vi "Example 2 Transient.vi"() -> ()   [LabVIEW 2015]
panel:
  out "time string 2":string
  out "time string":string
  in  "RANDOM":bool
  out "size(s)":i32
  out "Numeric":i32
  in  "Tab Control":enum32{"Page 1", "Page 2"}(tab)
  in  "no":bool
  in  "yes":bool
  in  "Memory SAVE":u16(ring)=3 items=["1", "2", "3", "4"]
  in  "message":string="Do you want store\n transient values"
  out "Model and SW rev,":string
  out "Array":string[](array[string])=["0,\"No error\""]
  in  "Tab Control 2":enum32{"INTERFACE", "TRANSIENT"}(tab)
  in  "Setting OK":bool
  in  "VISA":refnum<visa-resource-name>="COM1"
  in  "Baud Rate":i32(ring)=3 items=["1200", "2400", "4800", "9600", "19200", "38400", "57600", "115200"]
  in  "Address":i16=6
  in  "Voltage Limit at start":dbl=1.0 format="%.4f"
  in  "Current Limit at start":dbl=1.0 format="%.4f"
  in  "Reset (T)":bool
  out "Communication":bool=TRUE
  out "Appl. Rev":string
  in  "SCALE x":i8(slide)=1 scale=1.0..5.0
  in  "Tab Control 3":enum32{"Page 1", "Page 2"}(tab)
  in  "Max Element":i32=12
  out "Time/Dwell string [S]":string="0.97,0.90,0.45,0.31,0.84,0.30,0.65,0.95,0.00,0.05,0.72,0.12\r\n"
  out "Value string":string="7.93,8.01,0.22,1.41,9.70,1.73,7.77,7.95,7.10,1.88,5.55,1.76\r\n"
  in  "Max Time":dbl=1.0
  in  "Max Value":dbl=10.0
  out "Triggering value":dbl=0.9353250304502314
  in  "Step &\nCounter":cluster{"Step":u16, "Counter":dbl}={"Step"=1, "Counter"=1.0} {"Counter" min=1.0 max=9999.0 step=1.0; "Step" items=["ONCE", "AUTO"]}
  in  "Continius":u16(ring) caption="Continues (Default:0)" items=["0", "1"]
  out "Condition Setting":bool=TRUE
  in  "MODE":T1 caption="Cluster 1" {"Trans Mode (None)" items=["NONE", "FIX", "LIST", "WAVE"]; "Mode (V/I)" items=["VOLTAGE", "CURRENT"]}
  in  "Values":T2={"Value string"="001.00,003.00,002.00,004.00,003.00", "Time/Dwell string [S]"="0.100,0.100,0.100,0.100,0.100", "Triggering value "=0.0}
  out "Error":string
  out "READ VALUE":dbl format="%.4f"
  in  "dt Resolution":dbl=0.025 min=0.0 max=1.0 step=0.001
  in  "INIT":bool
  in  "Read SET/MEAS":bool=TRUE
  in  "ABORT":bool
  out "Waveform Graph":dynamicdata(graph)=[{"t0"=timestamp(0 s since 1904-01-01), "dt"=1.0, "Y"=[-0.05, -0.05, -0.05, -0.05, -0.05]}, {"t0"=timestamp(0 s since 1904-01-01), "dt"=0.02, "Y"=[7.81, 7.81, 7.81, 7.81, 7.81, 7.81, 7.81, 7.81, 7.81, 7.81, 7.81, 7.81, 7.81, 7.81, 7.81, 7.81, 7.81, 7.81, 7.81, 7.81, 7.81, 7.81, 7.81, 7.81, 7.81, 7.81, 7.81, 7.81, 7.81, 7.81, 7.81, 7.81, 7.81, 7.81, 7.81, 7.81, 7.81, 7.81, 7.81, 7.81, 7.81, 7.81, 7.81, 7.81, 7.81, 7.81, 7.81, 7.81, 7.81, 7.81, 7.81, 7.81, 7.81, 7.81, 7.81, 7.81, 7.81, 7.81, 7.81, 7.81, 7.81, 7.81, 7.81, 7.81, 7.81, 7.81, 7.81, 7.81, 7.81, 7.81, 7.81, 7.81, 7.81, 7.81, 7.81, 7.81, 7.81, 7.81, 7.81, 7.81, 7.81, 7.81, 7.81, 7.81, 7.81, 7.81, 7.81, 7.81, 7.81, 7.81, 7.81, 7.81, 7.81, 7.81, 7.81, 7.81, 7.81, 7.81, 7.81, 7.81, 7.81, 7.81, 7.81, 7.81, 7.81, 7.81, 7.81, 7.81, 7.81, 7.81, 7.81, 7.81, 7.81, 7.81, 7.81, 7.81, 7.81, 7.81, 7.81, 7.81, 7.81, 7.81, 7.81, 7.81, 7.81, 7.81, 7.81, 7.81, 7.81, 7.81, 7.81, 7.81, 7.81, 7.81, 7.81, 7.81, 7.81, 7.81, 7.81, 7.81, 7.81, 7.81, 7.81, 7.81, 7.81, 7.81, 7.81, 7.81, 7.81, 7.81, 7.81, 7.81, 7.81, 7.81, 7.81, 7.81, 7.81, 7.81, 7.81, 7.81, 7.81, 7.81, 7.81, 7.81, 7.81, 7.81, 7.81, 7.81, 7.81, 7.81, 7.81, 7.81, 7.81, 7.81, 7.81, 7.81, 7.81, 7.81, 7.81, 7.81]}]
  in  "Trig":bool
  in  "stop":bool
  in  "LOAD":enum32{"1", "2", "3", "4"}(radio)
  in  "STORe":enum32{"1", "2", "3", "4"}(radio)
  out "error out":errorcluster
  # "Configurate transient\nparameters"
  # "Z+ POWER SUPPLY"
  # "Set required interface and output parameters."
  # "PS Communication Language - SCPI"
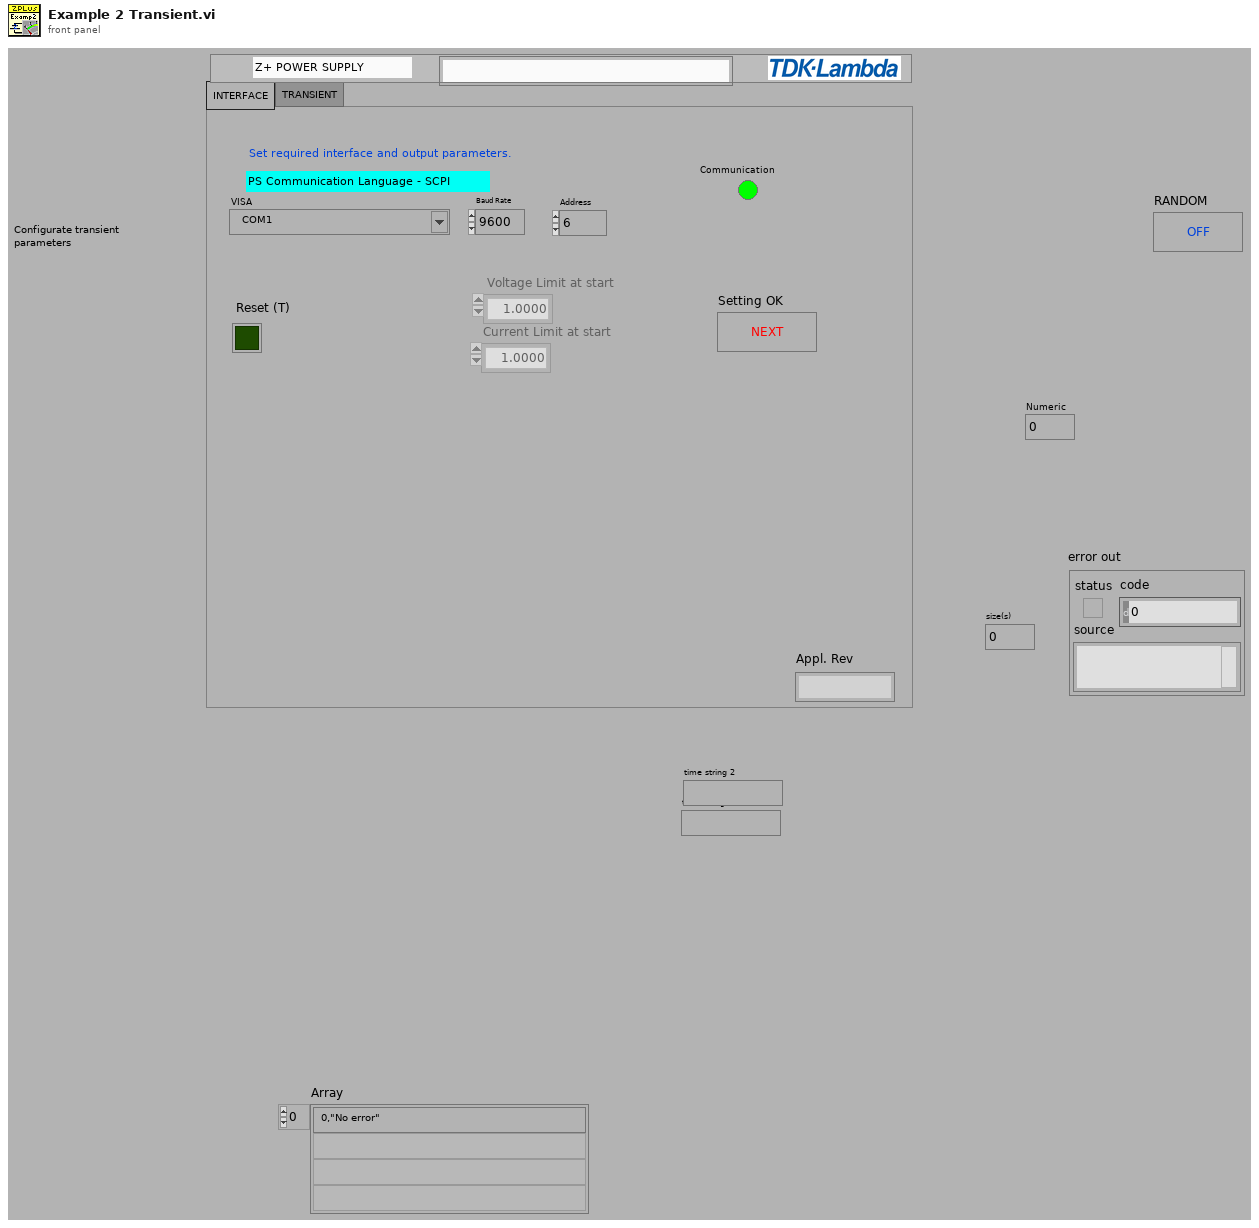
[diagram p1: front panel]
types:
  T1 = cluster{"Mode (V/I)":u16, "Trans Mode (None)":u16}
  T2 = cluster{"Value string":string, "Time/Dwell string [S]":string, "Triggering value ":dbl}
  T3 = enum8{"Enabled", "Disabled", "Disabled and Grayed Out"}
  T4 = cluster{"Response":string, "Response":string, "Triggering value (for fix)":dbl}
  T5 = cluster{"Value string":bool, "Time/Dwell string [S]":bool, "Triggering value ":bool}
  T6 = cluster{"Mode (V/I)":bool, "Trans Mode (None)":bool}
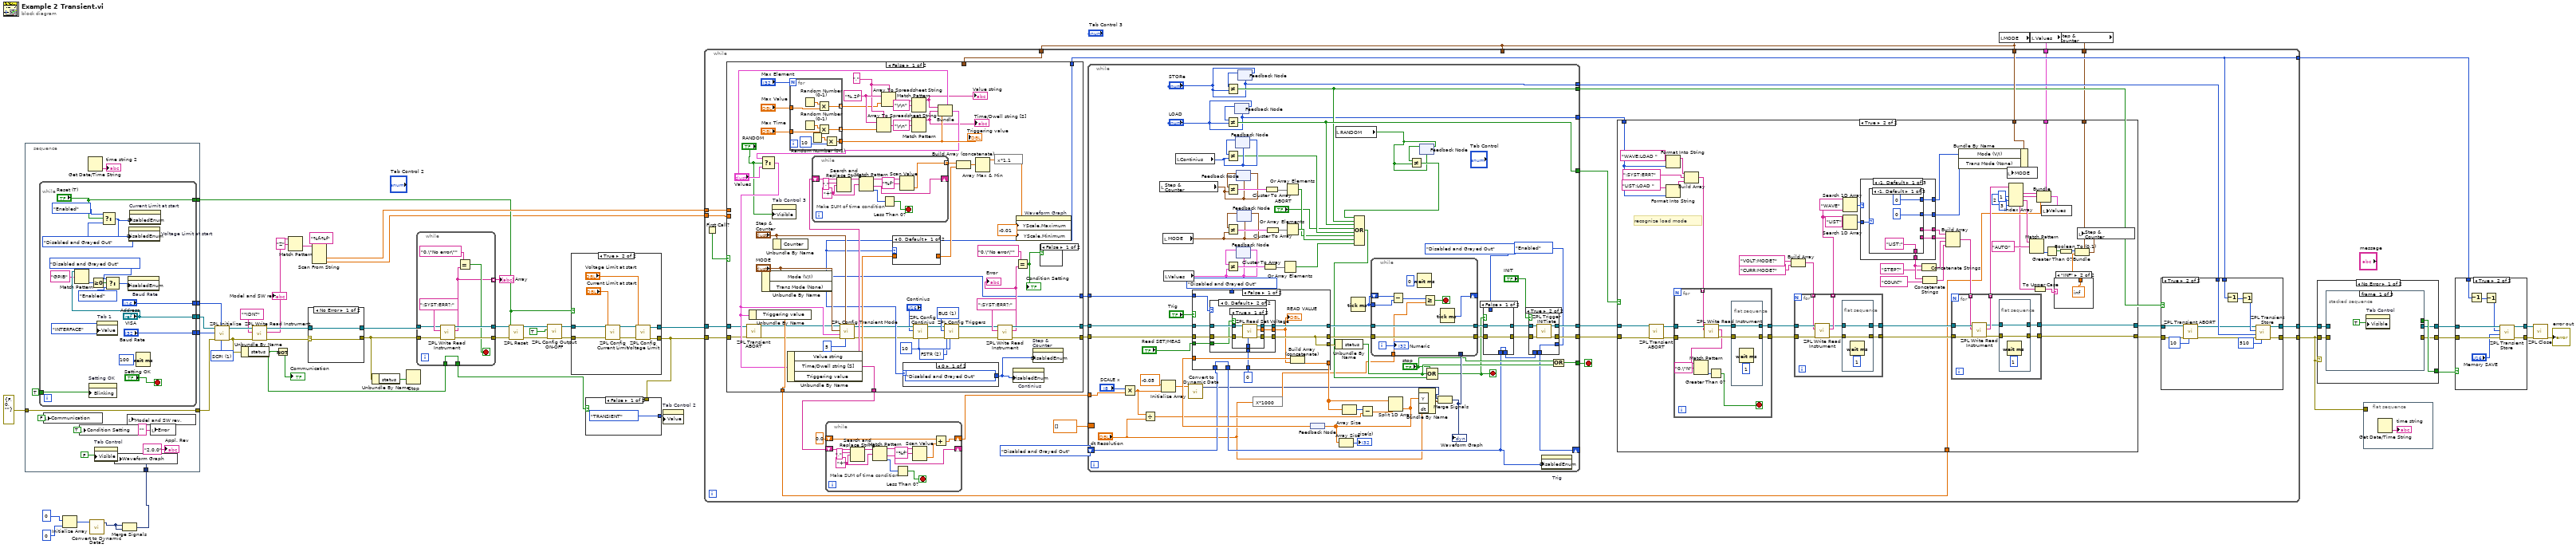
[diagram p0: block diagram]
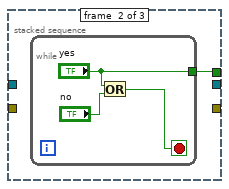
[diagram p3: hidden frame]
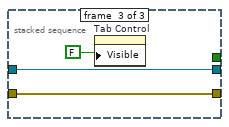
[diagram p4: hidden frame]
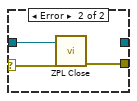
[diagram p6: hidden frame]
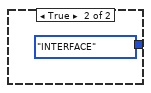
[diagram p7: hidden frame]
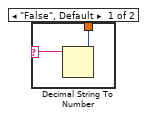
[diagram p11: hidden frame]
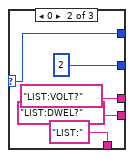
[diagram p12: hidden frame]
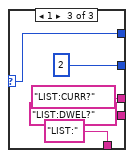
[diagram p13: hidden frame]
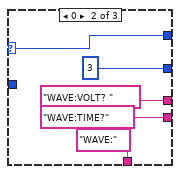
[diagram p14: hidden frame]
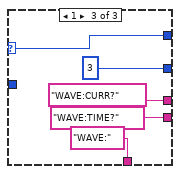
[diagram p15: hidden frame]
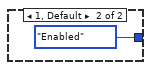
[diagram p17: hidden frame]
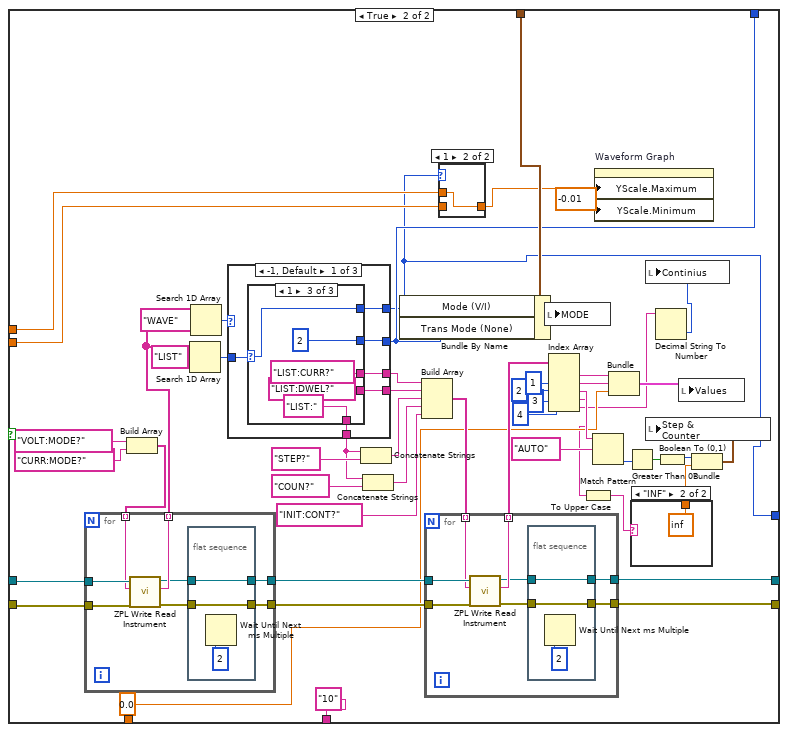
[diagram p19: hidden frame]
diagram:
  w18 = i16 1 items=["GEN", "SCPI"] ("Language Selector")
  n1 = Initialize Array(0 ("Read Set Voltage"), 0 ("dimension size")) -> (w7:i32[])
  n2 = call "Convert to Dynamic Data2"("Array"=w7) -> ("Dynamic Data Type"=w4:dynamicdata)  [unwired: 3 in]
  n3 = Merge Signals(w4, w4) -> (w3:dynamicdata)
  n4 = stacked-sequence {
    tunnel: [w58] -> w44
    tunnel: errorcluster {"status"=FALSE, "code"=0, "source"=""} ("error in") -> [w58]
    tunnel: [w62] -> w30
    tunnel: [w63] -> w29
    tunnel: [w64] -> w28
    tunnel: [w57] -> w15
    tunnel: w3 -> [w54]
    frame #0 {
      w56 = "" ("Response")
      n5 = while {
        tunnel: TRUE ("status") -> [w80]
        tunnel: ["Address"] -> w64
        tunnel: ["VISA"] -> w63
        tunnel: ["Baud Rate"] -> w62
        tunnel: ["Reset (T)"] -> w57
        stop <- "Setting OK" stop-if-true
        n6 = Match Pattern(string="VISA", regular expression="GPIB") -> (offset past match=w73:i32)  [unwired: 1 in, 3 out]
        n7 = property on="Setting OK" class="Bool"("Blinking"=w80) -> ()  [unwired: 2 in, 2 out]
        n8 = Greater Or Equal To 0?(x=w73) -> (x >= 0?=w74:bool)
        n9 = property on="Tab 1" class="TabCtl (strict)"("Value"=enum32{"INTERFACE", "TRANSIENT"}."INTERFACE" ("Tab Control 2")) -> ()  [unwired: 2 in, 2 out]
        n10 = Select(t=T3."Enabled" ("Disabled"), s="Reset (T)", f=T3."Disabled and Grayed Out" ("Disabled")) -> (s? t:f=w67:T3)
        n11 = Select(t=T3."Disabled and Grayed Out" ("Disabled"), s=w74, f=T3."Enabled" ("Disabled")) -> (s? t:f=w75:T3)
        n12 = property on="Baud Rate" class="Ring (strict)"("DisabledEnum"=w75) -> ()  [unwired: 2 in, 2 out]
        n13 = property on="Voltage Limit at start" class="DigNum (strict)"("DisabledEnum"=w67) -> ()  [unwired: 2 in, 2 out]
        n14 = property on="Current Limit at start" class="DigNum (strict)"("DisabledEnum"=w67) -> ()  [unwired: 2 in, 2 out]
        n15 = Wait (ms)(milliseconds to wait=u32 100) -> ()  [unwired: 1 out]
      }
      n16 = local write "Communication"(FALSE ("Communication")) -> ()
      n17 = local write "Condition Setting"(TRUE ("Condition Setting")) -> ()
      n18 = Get Date/Time String() -> (time string=→"time string 2":string)  [unwired: 3 in, 1 out]
      n19 = property on="Tab Control" class="TabCtl (strict)"("Visible"=FALSE) -> ()  [unwired: 2 in, 2 out]
      n20 = local write "Waveform Graph"(w54) -> ()
      n21 = local write "Model and SW rev,"(w56) -> ()
      n22 = local write "Error"(w56) -> ()
      "Appl. Rev" <- "2.0.0" ("rev")
    }
  }
  n23 = call "ZPL Initialize.vi"("Language Selector"=w18, "Address"=w28, "error in"=w44, "Baud Rate"=w30, "VISA"=w29) -> ("error out"=w38:errorcluster, "VISA  out"=w39:refnum<visa-resource-name>)  [unwired: 3 in, 2 out]
  n24 = Unbundle By Name(w38) -> ("status"=w8:bool)
  n25 = call "ZPL Write Read Instrument.vi"("error in"=w38, "Write Command/Query SCPI"="*IDN?", "VISA"=w39) -> ("error out"=w36:errorcluster, "Response"=w25:string, "VISA  out"=w35:refnum<visa-resource-name>)  [unwired: 6 in]
  "Model and SW rev," <- w25
  n26 = Not(x=w8) -> (.not. x?=→"Communication":bool)
  n27 = Match Pattern(string=w25, regular expression="Z") -> (after substring=w26:string)  [unwired: 1 in, 3 out]
  n28 = case shown="No Error" w36 {
    selector: w36 -> [w83 w87]
    tunnel: [w83 w86] -> w12
    tunnel: w35 -> [w84 w85]
    tunnel: [w84 _] -> w13
    frame No Error {
    }
    frame Error {
      n29 = call "ZPL Close.vi"("error"=w87, "VISA name"=w85) -> ("error out"=w86:errorcluster)  [unwired: 7 in]
    }
  }
  n30 = Scan From String(format string="%f-%f", input string=w26) -> (output 1=w23:dbl, output 2=w1:dbl)  [unwired: 4 in, 3 out]
  n31 = Unbundle By Name(w12) -> ("status"=w34:bool)
  n32 = Stop(stop? (T)=w34) -> ()
  n33 = while {
    tunnel: w13 -> [w94]
    tunnel: w12 -> [w93]
    tunnel: [w92] -> w33
    tunnel: [w91] -> w32
    tunnel: [w89] -> w31 mode=indexing
    tunnel: w8 -> [w88]
    tunnel: [w88] -> w10
    stop <- w90 stop-if-true
    n34 = call "ZPL Write Read Instrument.vi"("error in"=w93, "Write Command/Query SCPI"=":SYST:ERR?;", "VISA"=w94) -> ("error out"=w91:errorcluster, "Response"=w89:string, "VISA  out"=w92:refnum<visa-resource-name>)  [unwired: 6 in]
    n35 = Equal?(x="0,\"No error\"", y=w89) -> (x = y?=w90:bool)
  }
  "Array" <- w31
  n36 = call "ZPL Reset.vi"("error"=w32, "Reset (T)"=w15, "VISA"=w33) -> ("error out"=w40:errorcluster, "VISA out"=w51:refnum<visa-resource-name>)  [unwired: 7 in]
  n37 = call "ZPL Config Output ON-OFF.vi"("error"=w40, "Output ON"=TRUE, "VISA"=w51) -> ("error out"=w19:errorcluster, "VISA out"=w20:refnum<visa-resource-name>)  [unwired: 7 in]
  n38 = case shown="True" w15 {
    tunnel: [w98 w106] -> w43
    tunnel: [w97 w105] -> w9
    tunnel: w20 -> [w98 w104]
    tunnel: w19 -> [w97 w103]
    frame False {
    }
    frame True {
      n39 = call "ZPL Config Current Limit.vi"("error"=w103, "Current Limit"="Current Limit at start", "VISA"=w104) -> ("error out"=w102:errorcluster, "VISA out"=w101:refnum<visa-resource-name>)  [unwired: 7 in]
      n40 = call "ZPL Config Voltage Limit.vi"("error"=w102, "Voltage Limit"="Voltage Limit at start", "VISA"=w101) -> ("error out"=w105:errorcluster, "VISA out"=w106:refnum<visa-resource-name>)  [unwired: 7 in]
    }
  }
  n41 = case shown="False" w10 {
    tunnel: [enum32{"INTERFACE", "TRANSIENT"}."TRANSIENT" ("Tab Control 2") enum32{"INTERFACE", "TRANSIENT"}."INTERFACE" ("Tab Control 2")] -> w42
    tunnel: w9 -> [_ _]
    frame False {
    }
    frame True {
    }
  }
  n42 = property on="Tab Control 2" class="TabCtl (strict)"("Value"=w42) -> ()  [unwired: 2 in, 2 out]
  n43 = local read "MODE"() -> (w14:T1)
  n44 = local read "Values"() -> (w17:T2)
  n45 = local read "Step &\nCounter"() -> (w16:cluster{"Step":u16, "Counter":dbl})
  n46 = while {
    tunnel: [w124] -> w48
    tunnel: [w123] -> w2
    tunnel: w43 -> [w137]
    tunnel: w9 -> [w136]
    tunnel: w23 -> [w130]
    tunnel: w14 -> [w127]
    tunnel: [w120] -> w22
    tunnel: w17 -> [w116]
    tunnel: w16 -> [w115]
    tunnel: w14 -> [_]
    tunnel: w14 -> [w113]
    tunnel: w1 -> [w110]
    stop <- w131 stop-if-true
    n47 = First Call?() -> (First Call?: T/F=w111:bool)
    n48 = case shown="False" w111 {
      tunnel: w137 -> [w290 w373]
      tunnel: w136 -> [w289 w372]
      tunnel: [w330 "10" ("Time/Dwell string [S]")] -> w135
      tunnel: [w325 w371] -> w134
      tunnel: [w324 w370] -> w133
      tunnel: [w312 w355] -> w132
      tunnel: [w311 w362] -> w120
      tunnel: w130 -> [_ w358]
      tunnel: [w315 w369] -> w117
      tunnel: w113 -> [_ w363]
      tunnel: w110 -> [_ w357]
      frame False {
        w281 = u16 2 items=["OFF", "TRIG", "FSTR"] ("Trigger Out Mode")
        w282 = u32 10 ("Settle (1 mS)")
        w285 = u16 1 items=["EXT", "BUS"] ("Trigger in  Source")
        w310 = "%.2f" ("format string")
        w307 = "," ("delimiter (Tab)")
        n49 = call "ZPL Transient ABORT.vi"("error"=w289, "VISA"=w290) -> ("error out"=w287:errorcluster, "VISA out"=w288:refnum<visa-resource-name>)  [unwired: 8 in]
        n50 = Unbundle By Name("MODE") -> ("Mode (V/I)"=w312:u16, "Trans Mode (None)"=w311:u16)
        n51 = property on="Tab Control 3" class="TabCtl (strict)"("Visible"="RANDOM") -> ()  [unwired: 2 in, 2 out]
        n52 = Unbundle By Name("Step &\nCounter") -> ()  [unwired: 1 out]
        n53 = for {
          N: "Max Element" -> [_]
          tunnel: "Max Value" -> [w340]
          tunnel: [w339] -> w306 mode=indexing
          tunnel: "Max Time" -> [w337]
          tunnel: [w336] -> w308 mode=indexing
          tunnel: [w333] -> w302
          n54 = Random Number (0-1)() -> (number: 0 to 1=w341:dbl)
          n55 = Random Number (0-1)() -> (number: 0 to 1=w338:dbl)
          n56 = Random Number (0-1)() -> (number: 0 to 1=w335:dbl)
          n57 = Multiply(x=w341, y=w340) -> (x*y=w339:dbl)
          n58 = Multiply(x=w338, y=w337) -> (x*y=w336:dbl)
          n59 = Multiply(x=w335, y=10 ("Numeric 2")) -> (x*y=w333:dbl)
        }
        "Triggering value" <- w302
        n60 = Array To Spreadsheet String(delimiter (Tab)=w307, array=w308, 3:w310) -> (spreadsheet string=w298:string)
        n61 = Array To Spreadsheet String(delimiter (Tab)=w307, array=w306, 3:w310) -> (spreadsheet string=w295:string)
        n62 = case shown="0" w311 {
          tunnel: [T3."Disabled and Grayed Out" ("Disabled") T3."Enabled" ("Disabled")] -> w279
          frame 0 {
          }
          frame 1, Default {
          }
        }
        n63 = Match Pattern(string=w295, regular expression="\r\n") -> (before substring=w294:string)  [unwired: 1 in, 3 out]
        "Value string" <- w294
        n64 = Match Pattern(string=w298, regular expression="\r\n") -> (before substring=w293:string)  [unwired: 1 in, 3 out]
        "Time/Dwell string [S]" <- w293
        n65 = Bundle(cluster="Values", "Value string"=w294, "Time/Dwell string [S]"=w293, "Triggering value"=w302) -> (w301:T2)
        n66 = Select(t=w301, s="RANDOM", f="Values") -> (s? t:f=w300:T2)
        n67 = Unbundle By Name(w300) -> ("Triggering value"=w315:dbl)
        n68 = Unbundle By Name(w300) -> ("Value string"=w328:string, "Time/Dwell string [S]"=w330:string, "Triggering value"=w317:dbl)
        n69 = while {
          shift-right: [w352] -> _
          shift-left: w328 -> [w351]
          tunnel: [w345] -> w319 mode=indexing
          stop <- w349 stop-if-true
          w346 = "+" ("search string")
          # "Make SUM of time condition"
          n70 = Search and Replace String(input string=w351, search string=",", replace string=w346) -> (result string=w353:string)  [unwired: 5 in, 3 out]
          n71 = Match Pattern(string=w353, regular expression=w346) -> (before substring=w347:string, after substring=w352:string, offset past match=w350:i32)  [unwired: 1 in, 1 out]
          n72 = Less Than 0?(x=w350) -> (x < 0?=w349:bool)
          n73 = Scan Value(string=w347, format string="%f") -> (value=w345:dbl)  [unwired: 1 in, 1 out]
        }
        n74 = call "ZPL Config Transient Mode.vi"("Settle (1 mS)"=u32 5, "Step & Counter"="Step &\nCounter", "error"=w287, "Values"=w300, "MODE"="MODE", "VISA"=w288) -> ("error out"=w291:errorcluster, "VISA out"=w292:refnum<visa-resource-name>)  [unwired: 4 in]
        n75 = case shown="0, Default" w311 {
          tunnel: [_ w344] -> w316
          tunnel: w317 -> [_ w344]
          frame 0, Default {
          }
          frame 1 {
          }
        }
        n76 = call "ZPL Config Continius.vi"("Settle (1 mS)"=w282, "error"=w291, "Continius (Default:0)"="Continius", "VISA"=w292) -> ("error out"=w283:errorcluster, "VISA out"=w284:refnum<visa-resource-name>)  [unwired: 6 in]
        n77 = call "ZPL Config Triggers.vi"("Settle (1 mS)"=w282, "error"=w283, "Trigger Out Mode"=w281, "Trigger in  Source"=w285, "VISA"=w284) -> ("error out"=w313:errorcluster, "VISA out"=w314:refnum<visa-resource-name>)  [unwired: 4 in, 1 out]
        n78 = Build Array (concatenate)(w319, w316) -> (w318:dbl[])
        n79 = Array Max & Min(array=w318) -> (max value=w327:dbl)  [unwired: 3 out]
        n80 = expression code="x*1.1"(w327) -> (w326:dbl)
        n81 = call "ZPL Write Read Instrument.vi"("error in"=w313, "Write Command/Query SCPI"=":SYST:ERR?;", "VISA"=w314) -> ("error out"=w324:errorcluster, "Response"=w323:string, "VISA  out"=w325:refnum<visa-resource-name>)  [unwired: 6 in]
        "Error" <- w323
        n82 = property on="Continius" class="Ring (strict)"("DisabledEnum"=w279) -> ()  [unwired: 2 in, 2 out]
        n83 = Equal?(x="0,\"No error\"", y=w323) -> (x = y?=w286:bool)
        "Condition Setting" <- w286
        n84 = property on="Waveform Graph" class="WFGraph (strict)"("YScale.Maximum"=w326, "YScale.Minimum"=-0.01 ("Y Scale.Range:Minimum")) -> ()  [unwired: 2 in, 2 out]
        n85 = property on="Step &\nCounter" class="Clust (strict)"("DisabledEnum"=w279) -> ()  [unwired: 2 in, 2 out]
        n86 = case shown="False" w286 {
          frame False {
          }
          frame True {
          }
        }
      }
      frame True {
        w369 = 0.0 ("Triggering value (for fix)")
        n87 = Build Array("VOLT:MODE?" ("initial string"), "CURR:MODE?" ("initial string")) -> (w376:string[])
        n88 = for {
          tunnel: w373 -> [w459]
          tunnel: w372 -> [w458]
          tunnel: [w454] -> w382
          tunnel: [w453] -> w383
          tunnel: w376 -> [w452] mode=indexing
          tunnel: [w457] -> w379 mode=indexing
          n89 = call "ZPL Write Read Instrument.vi"("error in"=w458, "Write Command/Query SCPI"=w452, "VISA"=w459) -> ("error out"=w455:errorcluster, "Response"=w457:string, "VISA  out"=w456:refnum<visa-resource-name>)  [unwired: 6 in]
          n90 = flat-sequence {
            tunnel: w456 -> [w462]
            tunnel: w455 -> [w461]
            tunnel: [w462] -> w454
            tunnel: [w461] -> w453
            frame #0 {
              n91 = Wait Until Next ms Multiple(millisecond multiple=u32 2) -> ()  [unwired: 1 out]
            }
          }
        }
        n92 = Search 1D Array(1D array=w379, element="LIST" ("initial string")) -> (index of element=w380:i32)  [unwired: 1 in]
        n93 = Search 1D Array(1D array=w379, element="WAVE" ("initial string")) -> (index of element=w381:i32)  [unwired: 1 in]
        n94 = case shown="-1, Default" w381 {
          selector: w381 -> [_ w442 w447]
          tunnel: w380 -> [w428 _ _]
          tunnel: [w427 w442 w447] -> w355
          tunnel: [w426 3 3] -> w362
          tunnel: [w425 "WAVE:VOLT? " ("initial string") "WAVE:CURR?" ("initial string")] -> w384
          tunnel: [w424 "WAVE:TIME?" ("initial string") "WAVE:TIME?" ("initial string")] -> w385
          tunnel: [w423 "WAVE:" ("initial string") "WAVE:" ("initial string")] -> w392
          frame -1, Default {
            n95 = case shown="1" w428 {
              selector: w428 -> [_ w433 w438]
              tunnel: [0 w433 w438] -> w427
              tunnel: [0 2 2] -> w426
              tunnel: [_ "LIST:VOLT?" ("initial string") "LIST:CURR?" ("initial string")] -> w425
              tunnel: [_ "LIST:DWEL?" ("initial string") "LIST:DWEL?" ("initial string")] -> w424
              tunnel: ["LIST:" ("initial string") "LIST:" ("initial string") "LIST:" ("initial string")] -> w423
              frame -1, Default {
              }
              frame 0 {
              }
              frame 1 {
              }
            }
          }
          frame 0 {
          }
          frame 1 {
          }
        }
        n96 = Concatenate Strings(w392, "STEP?" ("string")) -> (w395:string)
        n97 = Concatenate Strings(w392, "COUN?" ("string")) -> (w396:string)
        n98 = Bundle By Name(cluster=w363, "Mode (V/I)"=w355, "Trans Mode (None)"=w362) -> (w364:T1)
        n99 = Build Array(w384, w385, w395, w396, "INIT:CONT?" ("string")) -> (w386:string[])
        n100 = for {
          tunnel: w382 -> [w419]
          tunnel: w383 -> [w418]
          tunnel: [w414] -> w371
          tunnel: [w413] -> w370
          tunnel: w386 -> [w412] mode=indexing
          tunnel: [w417] -> w387 mode=indexing
          n101 = call "ZPL Write Read Instrument.vi"("error in"=w418, "Write Command/Query SCPI"=w412, "VISA"=w419) -> ("error out"=w415:errorcluster, "Response"=w417:string, "VISA  out"=w416:refnum<visa-resource-name>)  [unwired: 6 in]
          n102 = flat-sequence {
            tunnel: w416 -> [w422]
            tunnel: w415 -> [w421]
            tunnel: [w422] -> w414
            tunnel: [w421] -> w413
            frame #0 {
              n103 = Wait Until Next ms Multiple(millisecond multiple=u32 2) -> ()  [unwired: 1 out]
            }
          }
        }
        n104 = case shown="1" w355 {
          tunnel: w358 -> [_ w408]
          tunnel: w357 -> [w407 _]
          tunnel: [w407 w408] -> w356
          frame 0, Default {
          }
          frame 1 {
          }
        }
        n105 = local write "MODE"(w364) -> ()
        n106 = Index Array(array=w387, index #2=1 ("index"), index #3=2 ("index"), index #4=3 ("index"), index #5=4 ("index")) -> (element #1=w390:string, element #2=w389:string, element #3=w401:string, element #4=w361:string, element #5=w366:string)  [unwired: 1 in]
        n107 = To Upper Case(1:w361) -> (0:w360:string)
        n108 = Match Pattern(string=w401, regular expression="AUTO") -> (offset past match=w403:i32)  [unwired: 1 in, 3 out]
        n109 = property on="Waveform Graph" class="WFGraph (strict)"("YScale.Maximum"=w356, "YScale.Minimum"=-0.01 ("Y Scale.Range:Minimum")) -> ()  [unwired: 2 in, 2 out]
        n110 = Bundle("Response"=w390, "Response"=w389, "Triggering value (for fix)"=w369) -> (w391:T4)  [unwired: 1 in]
        n111 = Greater Than 0?(x=w403) -> (x > 0?=w404:bool)
        n112 = case shown="\"INF\"" w360 {
          selector: w360 -> [w409 _]
          tunnel: [w410 inf] -> w400
          frame "False", Default {
            n113 = Decimal String To Number(string=w409) -> (number=w410:i32)  [unwired: 2 in, 1 out]
          }
          frame "INF" {
          }
        }
        n114 = Decimal String To Number(string=w366) -> (number=w365:i32)  [unwired: 2 in, 1 out]
        n115 = local write "Continius"(w365) -> ()
        n116 = Boolean To (0,1)(Boolean=w404) -> (0, 1=w405:i16)
        n117 = local write "Values"(w391) -> ()
        n118 = Bundle(w405, w400) -> (w399:cluster{i16, dbl})  [unwired: 1 in]
        n119 = local write "Step &\nCounter"(w399) -> ()
      }
    }
    n120 = while {
      shift-right: [w472] -> _
      shift-left: w135 -> [w471]
      shift-right: [w465] -> w112
      shift-left: 0.0 -> [w464]
      stop <- w469 stop-if-true
      w463 = "+" ("search string")
      # "Make SUM of time condition"
      n121 = Search and Replace String(input string=w471, search string=",", replace string=w463) -> (result string=w473:string)  [unwired: 5 in, 3 out]
      n122 = Match Pattern(string=w473, regular expression=w463) -> (before substring=w467:string, after substring=w472:string, offset past match=w470:i32)  [unwired: 1 in, 1 out]
      n123 = Less Than 0?(x=w470) -> (x < 0?=w469:bool)
      n124 = Scan Value(string=w467, format string="%f") -> (value=w466:dbl)  [unwired: 1 in, 1 out]
      n125 = Add(x=w464, y=w466) -> (x+y=w465:dbl)
    }
    n126 = while {
      tunnel: w134 -> [w548]
      tunnel: w133 -> [w547]
      tunnel: [w500] -> w129
      tunnel: [w499] -> w128
      tunnel: [w507] -> w131
      tunnel: w132 -> [w511]
      tunnel: ["LOAD"] -> w126
      tunnel: [w505] -> w125
      tunnel: ["STORe"] -> w118
      tunnel: [w503] -> w119
      shift-right: [w493] -> _
      shift-left: T3."Disabled and Grayed Out" ("Disabled") -> [w485]
      tunnel: w112 -> [w477]
      border: dbl[] [] -> [_]
      stop <- w497 stop-if-true
      n127 = Multiply(x="SCALE x", y=w477) -> (x*y=w475:dbl)
      n128 = Divide(x=w475, y="dt Resolution") -> (x/y=w478:dbl)
      n129 = local read "Step &\nCounter"() -> (w522:cluster{"Step":u16, "Counter":dbl})
      n130 = Initialize Array(-0.05 ("Read Set Voltage"), w475) -> (w482:dbl[])
      n131 = local read "MODE"() -> (w527:T1)
      n132 = local read "Values"() -> (w526:T2)
      n133 = local read "Continius"() -> (w519:u16)
      n134 = call "Convert to Dynamic Data"("Array"=w482) -> ("Dynamic Data Type"=w480:dynamicdata)  [unwired: 3 in]
      n135 = feedback-in #1("LOAD") -> ()
      n136 = feedback #1("LOAD") -> (w506:enum32{"1", "2", "3", "4"})
      n137 = Not Equal?(x=w506, y="LOAD") -> (x != y?=w505:bool)
      n138 = feedback-in #2(w519) -> ()
      n139 = feedback #2(w519) -> (w520:u16)
      n140 = Not Equal?(x=w520, y=w519) -> (x != y?=w518:bool)
      n141 = feedback-in #3(w526) -> ()
      n142 = feedback #3(w526) -> (w531:T2)
      n143 = Not Equal?(x=w531, y=w526) -> (x != y?=w532:T5)
      n144 = feedback-in #4(w522) -> ()
      n145 = feedback #4(w522) -> (w523:cluster{"Step":u16, "Counter":dbl})
      n146 = Not Equal?(x=w523, y=w522) -> (x != y?=w524:cluster{"Step":bool, "Counter":bool})
      n147 = feedback-in #5(w527) -> ()
      n148 = feedback #5(w527) -> (w534:T1)
      n149 = Not Equal?(x=w534, y=w527) -> (x != y?=w535:T6)
      n150 = feedback-in #6("STORe") -> ()
      n151 = feedback #6("STORe") -> (w504:enum32{"1", "2", "3", "4"})
      n152 = Not Equal?(x=w504, y="STORe") -> (x != y?=w503:bool)
      n153 = expression code="X*1000"("dt Resolution") -> (w489:dbl)
      n154 = Cluster To Array(cluster=w532) -> (array=w533:bool[])
      n155 = Cluster To Array(cluster=w524) -> (array=w525:bool[])
      n156 = Cluster To Array(cluster=w535) -> (array=w536:bool[])
      n157 = Or Array Elements(Boolean array=w533) -> (logical OR=w530:bool)
      n158 = Or Array Elements(Boolean array=w525) -> (logical OR=w521:bool)
      n159 = Or Array Elements(Boolean array=w536) -> (logical OR=w529:bool)
      n160 = feedback #7() -> (w544:dbl[])
      n161 = case shown="False" "Trig" {
        tunnel: w548 -> [w585 w630]
        tunnel: w547 -> [w584 w629]
        tunnel: [w583 w632] -> w542
        tunnel: [w582 w631] -> w543
        tunnel: [w582 w631] -> w545
        tunnel: w544 -> [w581 w628]
        tunnel: [w580 w628] -> w539
        tunnel: u32 0 ("Settle (1 mS)") -> [w578 _]
        tunnel: w511 -> [w577 _]
        tunnel: "Read SET/MEAS" -> [w576 _]
        tunnel: w485 -> [w575 w626]
        tunnel: [w575 w625] -> w484
        tunnel: T3."Disabled and Grayed Out" ("Disabled") -> [_ w624]
        frame False {
          n162 = case shown="0, Default" w577 {
            tunnel: w585 -> [w592 w611]
            tunnel: w584 -> [w591 w610]
            tunnel: [w590 w609] -> w583
            tunnel: [w589 w608] -> w582
            tunnel: [w588 w607] -> w579
            tunnel: w578 -> [w587 w606]
            tunnel: w576 -> [w586 w605]
            frame 1 {
              n163 = case shown="True" w586 {
                tunnel: w592 -> [w598 w604]
                tunnel: w591 -> [w597 w603]
                tunnel: [w596 w602] -> w590
                tunnel: [w595 w601] -> w589
                tunnel: [w594 w600] -> w588
                tunnel: w587 -> [w593 w599]
                frame True {
                  n164 = call "ZPL Read Set Current.vi"("Settle (1 mS)"=w593, "error"=w597, "VISA"=w598) -> ("error out"=w595:errorcluster, "Read Set Current"=w594:dbl, "VISA out"=w596:refnum<visa-resource-name>)  [unwired: 6 in]
                }
                frame False {
                  n165 = call "ZPL Meas Output Current.vi"("Settle (1 mS)"=w599, "error"=w603, "VISA"=w604) -> ("error out"=w601:errorcluster, "Output Current"=w600:dbl, "VISA out"=w602:refnum<visa-resource-name>)  [unwired: 6 in]
                }
              }
            }
            frame 0, Default {
              n166 = case shown="True" w605 {
                tunnel: w611 -> [w617 w623]
                tunnel: w610 -> [w616 w622]
                tunnel: [w615 w621] -> w609
                tunnel: [w614 w620] -> w608
                tunnel: [w613 w619] -> w607
                tunnel: w606 -> [w612 w618]
                frame True {
                  n167 = call "ZPL Read Set Voltage.vi"("Settle (1 mS)"=w612, "error"=w616, "VISA"=w617) -> ("error out"=w614:errorcluster, "Read Set Voltage"=w613:dbl, "VISA out"=w615:refnum<visa-resource-name>)  [unwired: 6 in]
                }
                frame False {
                  n168 = call "ZPL Meas Output Voltage.vi"("Settle (1 mS)"=w618, "error"=w622, "VISA"=w623) -> ("error out"=w620:errorcluster, "Output Voltage"=w619:dbl, "VISA out"=w621:refnum<visa-resource-name>)  [unwired: 6 in]
                }
              }
            }
          }
          "READ VALUE" <- w579
          n169 = Build Array (concatenate)(w581, w579) -> (w580:dbl[])
        }
        frame True {
          n170 = local read "Continius"() -> (w627:u16)
          n171 = case shown="0, Default" w627 {
            tunnel: w626 -> [_ w634]
            tunnel: [w633 w634] -> w625
            tunnel: w624 -> [w633 _]
            frame 0, Default {
            }
            frame 1 {
            }
          }
          n172 = call "ZPL Trigger.vi"("error"=w629, "VISA"=w630) -> ("error out"=w631:errorcluster, "VISA out"=w632:refnum<visa-resource-name>)  [unwired: 8 in]
        }
      }
      n173 = Unbundle By Name(w545) -> ("status"=w509:bool)
      n174 = local read "RANDOM"() -> (w490:bool)
      n175 = Array Size(array=w539) -> (size(s)=w538:i32)
      n176 = Tick Count (ms)() -> (millisecond timer value=w541:u32)
      n177 = Subtract(x=w538, y=w478) -> (x-y=w537:dbl)
      n178 = Split 1D Array(array=w539, index=w537) -> (second subarray=w517:dbl[])  [unwired: 1 out]
      n179 = feedback-in #7(w517) -> ()
      n180 = Array Size(array=w517) -> (size(s)=→"size(s)":i32)
      n181 = Bundle By Name("Y"=w517, "dt"="dt Resolution") -> (w540:waveform(dbl))  [unwired: 1 in]
      n182 = feedback-in #8(w490) -> ()
      n183 = feedback #8(w490) -> (w492:bool)
      n184 = Not Equal?(x=w492, y=w490) -> (x != y?=w491:bool)
      n185 = Compound Arithmetic op=OR(w491, w503, w505, "ABORT", w518, w521, w529, w530) -> (w528:bool)
      n186 = Compound Arithmetic op=OR("stop", w509, w528) -> (w497:bool)
      n187 = Merge Signals(w480, w540) -> (w516:dynamicdata)
      "Waveform Graph" <- w516
      n188 = while {
        tunnel: w543 -> [w558]
        tunnel: w542 -> [w557]
        tunnel: [w558] -> w514
        tunnel: [w557] -> w515
        shift-right: [w554] -> _
        shift-left: w541 -> [w552]
        tunnel: w541 -> [w553]
        tunnel: w516 -> [_]
        tunnel: w489 -> [w549]
        i -> [w551]
        stop <- w555 stop-if-true
        n189 = Subtract(x=w552, y=w553) -> (x-y=w556:u32)
        n190 = Wait (ms)(milliseconds to wait=u32 0) -> ()  [unwired: 1 out]
        n191 = Greater Or Equal?(x=w556, y=w549) -> (x >= y?=w555:bool)
        n192 = Tick Count (ms)() -> (millisecond timer value=w554:u32)
        "Numeric" <- w551
      }
      n193 = case shown="False" w497 {
        tunnel: w515 -> [w569 w573]
        tunnel: w514 -> [w568 w572]
        tunnel: [w569 w571] -> w502
        tunnel: [w568 w570] -> w501
        tunnel: w484 -> [w567 _]
        tunnel: [w567 w574] -> w496
        tunnel: T3."Disabled and Grayed Out" ("Disabled") -> [_ w574]
        frame False {
        }
        frame True {
          n194 = call "ZPL Transient ABORT.vi"("error"=w572, "VISA"=w573) -> ("error out"=w570:errorcluster, "VISA out"=w571:refnum<visa-resource-name>)  [unwired: 8 in]
        }
      }
      n195 = case shown="True" "INIT" {
        tunnel: w502 -> [w561 w566]
        tunnel: w501 -> [w560 w565]
        tunnel: [w561 w564] -> w500
        tunnel: [w560 w563] -> w499
        tunnel: w496 -> [w559 _]
        tunnel: [w559 w562] -> w493
        tunnel: T3."Enabled" ("Disabled") -> [_ w562]
        frame False {
        }
        frame True {
          n196 = call "ZPL Trigger INITiate.vi"("error"=w565, "VISA"=w566) -> ("error out"=w563:errorcluster, "VISA out"=w564:refnum<visa-resource-name>)  [unwired: 8 in]
        }
      }
      n197 = property on="Trig" class="Bool"("DisabledEnum"=w484) -> ()  [unwired: 2 in, 2 out]
      n198 = Compound Arithmetic op=OR("stop", w509) -> (w507:bool)
    }
    n199 = case shown="True" w125 {
      tunnel: w129 -> [w154 w210]
      tunnel: w128 -> [w153 w209]
      tunnel: [w154 w159] -> w122
      tunnel: [w153 w158] -> w121
      tunnel: w127 -> [_ w196]
      tunnel: w126 -> [_ w166]
      tunnel: w117 -> [_ w172]
      tunnel: w116 -> [_ w161]
      tunnel: w115 -> [_ w160]
      frame False {
      }
      frame True {
        # "recognize load mode"
        n200 = call "ZPL Transient ABORT.vi"("error"=w209, "VISA"=w210) -> ("error out"=w170:errorcluster, "VISA out"=w171:refnum<visa-resource-name>)  [unwired: 8 in]
        n201 = Format Into String(initial string="WAVE:LOAD ", w166) -> (resulting string=w164:string)  [unwired: 2 in, 1 out]
        n202 = Format Into String(initial string="LIST:LOAD ", w166) -> (resulting string=w165:string)  [unwired: 2 in, 1 out]
        n203 = Build Array(w164, ":SYST:ERR?" ("Write Command/Query SCPI"), w165) -> (w162:string[])
        n204 = for {
          tunnel: w171 -> [w224]
          tunnel: w170 -> [w223]
          tunnel: [w220] -> w169
          tunnel: [w219] -> w168
          tunnel: w162 -> [w218] mode=indexing
          stop <- w214 stop-if-true
          n205 = call "ZPL Write Read Instrument.vi"("error in"=w223, "Write Command/Query SCPI"=w218, "VISA"=w224) -> ("error out"=w221:errorcluster, "Response"=w216:string, "VISA  out"=w222:refnum<visa-resource-name>)  [unwired: 6 in]
          n206 = Match Pattern(string=w216, regular expression="0,\"N") -> (offset past match=w215:i32)  [unwired: 1 in, 3 out]
          n207 = Greater Than 0?(x=w215) -> (x > 0?=w214:bool)
          n208 = flat-sequence {
            tunnel: w222 -> [w227]
            tunnel: w221 -> [w226]
            tunnel: [w227] -> w220
            tunnel: [w226] -> w219
            frame #0 {
              n209 = Wait (ms)(milliseconds to wait=u32 1 ("millisecond multiple")) -> ()  [unwired: 1 out]
            }
          }
        }
        n210 = Build Array("VOLT:MODE?" ("initial string"), "CURR:MODE?" ("initial string")) -> (w205:string[])
        n211 = for {
          tunnel: w169 -> [w275]
          tunnel: w168 -> [w274]
          tunnel: [w270] -> w195
          tunnel: [w269] -> w194
          tunnel: w205 -> [w268] mode=indexing
          tunnel: [w273] -> w202 mode=indexing
          n212 = call "ZPL Write Read Instrument.vi"("error in"=w274, "Write Command/Query SCPI"=w268, "VISA"=w275) -> ("error out"=w271:errorcluster, "Response"=w273:string, "VISA  out"=w272:refnum<visa-resource-name>)  [unwired: 6 in]
          n213 = flat-sequence {
            tunnel: w272 -> [w278]
            tunnel: w271 -> [w277]
            tunnel: [w278] -> w270
            tunnel: [w277] -> w269
            frame #0 {
              n214 = Wait (ms)(milliseconds to wait=u32 1 ("millisecond multiple")) -> ()  [unwired: 1 out]
            }
          }
        }
        n215 = Search 1D Array(1D array=w202, element="LIST" ("initial string")) -> (index of element=w201:i32)  [unwired: 1 in]
        n216 = Search 1D Array(1D array=w202, element="WAVE" ("initial string")) -> (index of element=w200:i32)  [unwired: 1 in]
        n217 = case shown="-1, Default" w200 {
          selector: w200 -> [_ w258 w263]
          tunnel: w201 -> [w244 _ _]
          tunnel: [w243 w258 w263] -> w198
          tunnel: [w242 3 3] -> w199
          tunnel: [w241 "WAVE:VOLT? " ("initial string") "WAVE:CURR?" ("initial string")] -> w193
          tunnel: [w240 "WAVE:TIME?" ("initial string") "WAVE:TIME?" ("initial string")] -> w192
          tunnel: [w239 "WAVE:" ("initial string") "WAVE:" ("initial string")] -> w185
          frame -1, Default {
            n218 = case shown="-1, Default" w244 {
              selector: w244 -> [_ w249 w254]
              tunnel: [0 w249 w254] -> w243
              tunnel: [0 2 2] -> w242
              tunnel: [_ "LIST:VOLT?" ("initial string") "LIST:CURR?" ("initial string")] -> w241
              tunnel: [_ "LIST:DWEL?" ("initial string") "LIST:DWEL?" ("initial string")] -> w240
              tunnel: ["LIST:" ("initial string") "LIST:" ("initial string") "LIST:" ("initial string")] -> w239
              frame -1, Default {
              }
              frame 0 {
              }
              frame 1 {
              }
            }
          }
          frame 0 {
          }
          frame 1 {
          }
        }
        n219 = Concatenate Strings(w185, "STEP?" ("string")) -> (w182:string)
        n220 = Concatenate Strings(w185, "COUN?" ("string")) -> (w181:string)
        n221 = Build Array(w193, w192, w182, w181) -> (w191:string[])
        n222 = for {
          tunnel: w195 -> [w235]
          tunnel: w194 -> [w234]
          tunnel: [w230] -> w159
          tunnel: [w229] -> w158
          tunnel: w191 -> [w228] mode=indexing
          tunnel: [w233] -> w190 mode=indexing
          n223 = call "ZPL Write Read Instrument.vi"("error in"=w234, "Write Command/Query SCPI"=w228, "VISA"=w235) -> ("error out"=w231:errorcluster, "Response"=w233:string, "VISA  out"=w232:refnum<visa-resource-name>)  [unwired: 6 in]
          n224 = flat-sequence {
            tunnel: w232 -> [w238]
            tunnel: w231 -> [w237]
            tunnel: [w238] -> w230
            tunnel: [w237] -> w229
            frame #0 {
              n225 = Wait (ms)(milliseconds to wait=u32 1 ("millisecond multiple")) -> ()  [unwired: 1 out]
            }
          }
        }
        n226 = Bundle By Name(cluster=w196, "Mode (V/I)"=w198, "Trans Mode (None)"=w199) -> (w197:T1)
        n227 = local write "MODE"(w197) -> ()
        n228 = Index Array(array=w190, index #2=1 ("index"), index #3=2 ("index"), index #4=3 ("index")) -> (element #1=w187:string, element #2=w188:string, element #3=w177:string, element #4=w157:string)  [unwired: 1 in]
        n229 = Match Pattern(string=w177, regular expression="AUTO") -> (offset past match=w175:i32)  [unwired: 1 in, 3 out]
        n230 = To Upper Case(1:w157) -> (0:w156:string)
        n231 = Bundle(cluster=w161, "Value string"=w187, "Time/Dwell string [S]"=w188, "Triggering value"=w172) -> (w186:T2)
        n232 = local write "Values"(w186) -> ()
        n233 = Greater Than 0?(x=w175) -> (x > 0?=w174:bool)
        n234 = case shown="\"INF\"" w156 {
          selector: w156 -> [w211 _]
          tunnel: [w212 inf] -> w155
          frame "False", Default {
            n235 = Decimal String To Number(string=w211) -> (number=w212:i32)  [unwired: 2 in, 1 out]
          }
          frame "INF" {
          }
        }
        n236 = Boolean To (0,1)(Boolean=w174) -> (0, 1=w173:i16)
        n237 = Bundle(cluster=w160, "Step"=w173, "Counter"=w155) -> (w178:cluster{"Step":u16, "Counter":dbl})
        n238 = local write "Step &\nCounter"(w178) -> ()
      }
    }
    n239 = case shown="True" w119 {
      tunnel: [w140 w152] -> w124
      tunnel: [w139 w151] -> w123
      tunnel: w122 -> [w140 w143]
      tunnel: w121 -> [w139 w144]
      tunnel: w120 -> [_ w150]
      tunnel: w118 -> [_ w147]
      frame False {
      }
      frame True {
        n240 = call "ZPL Transient ABORT.vi"("Settle (1 mS)"=u32 10, "error"=w144, "VISA"=w143) -> ("error out"=w141:errorcluster, "VISA out"=w142:refnum<visa-resource-name>)  [unwired: 7 in]
        n241 = Decrement(x=w150) -> (x-1=w148:i32)
        n242 = Decrement(x=w148) -> (x-1=w149:i32)
        n243 = call "ZPL Transient Store.vi"("Settle (1 mS)"=u32 510, "error"=w141, "Memory SAVE"=w147, "Save Mode"=w149, "VISA"=w142) -> ("error out"=w151:errorcluster, "VISA out"=w152:refnum<visa-resource-name>)  [unwired: 5 in]
      }
    }
  }
  n244 = case shown="No Error" w2 {
    tunnel: w48 -> [w639 w649]
    tunnel: w2 -> [w638 w648]
    tunnel: [w637 _] -> w47
    tunnel: [w636 w649] -> w46
    tunnel: [w635 w648] -> w45
    frame No Error {
      n245 = stacked-sequence {
        tunnel: w639 -> [_ _ w646]
        tunnel: w638 -> [_ _ w645]
        tunnel: [_ w641 _] -> w637
        tunnel: [_ _ w646] -> w636
        tunnel: [_ _ w645] -> w635
        frame #0 {
          n246 = property on="Tab Control" class="TabCtl (strict)"("Visible"=TRUE) -> ()  [unwired: 2 in, 2 out]
        }
        frame #1 {
          n247 = while {
            tunnel: ["yes"] -> w641
            stop <- w642 stop-if-true
            n248 = Or(x="yes", y="no") -> (x .or. y?=w642:bool)
          }
        }
        frame #2 {
          n249 = property on="Tab Control" class="TabCtl (strict)"("Visible"=FALSE) -> ()  [unwired: 2 in, 2 out]
        }
      }
    }
    frame Error {
    }
  }
  n250 = flat-sequence {
    tunnel: w2 -> [_]
    frame #0 {
      n251 = Get Date/Time String() -> (time string=→"time string":string)  [unwired: 3 in, 1 out]
    }
  }
  n252 = case shown="True" w47 {
    tunnel: [w652 w660] -> w50
    tunnel: [w651 w659] -> w49
    tunnel: w46 -> [w652 w658]
    tunnel: w45 -> [w651 w657]
    tunnel: w22 -> [_ w656]
    frame False {
    }
    frame True {
      n253 = Decrement(x=w656) -> (x-1=w654:i32)
      n254 = Decrement(x=w654) -> (x-1=w655:i32)
      n255 = call "ZPL Transient Store.vi"("error"=w657, "Memory SAVE"="Memory SAVE", "Save Mode"=w655, "VISA"=w658) -> ("error out"=w659:errorcluster, "VISA out"=w660:refnum<visa-resource-name>)  [unwired: 6 in]
    }
  }
  n256 = call "ZPL Close.vi"("error"=w49, "VISA name"=w50) -> ("error out"=→"error out":errorcluster)  [unwired: 7 in]
